vi "WinCI Get Default Provider.vi"(8 "error in (no error)":errorcluster) -> (0 "error out":errorcluster, 2 "default provider":string)   [LabVIEW 2017, in "NI_SCC_WinCI.lvlib"]
uses:
  <vilib>/SourceControl/Providers/WinCI/NI_SCC_WinCI.lvlib
  <vilib>/registry/registry.llb/Registry RtKey.ctl
  <vilib>/registry/registry.llb/Registry SAM.ctl
  <vilib>/registry/registry.llb/Read Registry Value Simple STR.vi
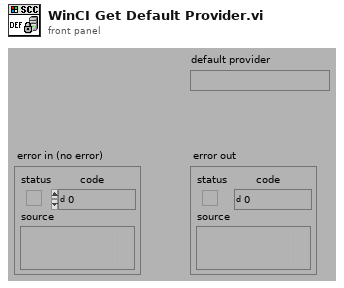
[diagram p1: front panel]
types:
  T1 = typedef "Registry SAM.ctl" = enum32{"KEY_QUERY_VALUE", "KEY_SET_VALUE", "KEY_CREATE_SUB_KEY", "KEY_ENUMERATE_SUB_KEYS", "KEY_NOTIFY", "KEY_CREATE_LINK", "KEY_READ", "KEY_WRITE", "KEY_ALL_ACCESS", "KEY_READ | KEY_WRITE"}
  T2 = typedef "Registry RtKey.ctl" = enum32{"HKEY_CLASSES_ROOT", "HKEY_CURRENT_USER", "HKEY_LOCAL_MACHINE", "HKEY_USERS", "HKEY_PERFORMANCE_DATA", "HKEY_CURRENT_CONFIG", "HKEY_DYN_DATA"}
  T3 = typedef "Registry refnum.ctl" = refnum<k1>
  T4 = cluster{"numValues":i32, "maxValueNameLen":i32, "maxValueDataLen":i32}
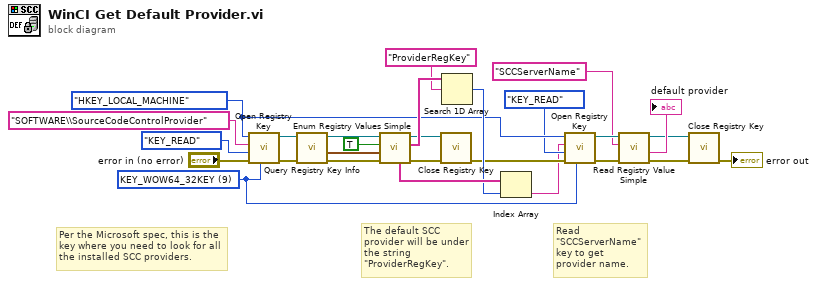
[diagram p0: block diagram]
diagram:
  w1 = u16 9 items=["DEFAULT"=0, "KEY_WOW64_64KEY"=8, "KEY_WOW64_32KEY"=9] ("alternate registry view mask")
  w9 = Registry_RtKey."HKEY_LOCAL_MACHINE" ("root key (HKEY_LOCAL_MACHINE)")
  # "Read \"SCCServerName\" key to get provider name."
  # "The default SCC provider will be under the string \"ProviderRegKey\"."
  # "Per the Microsoft spec, this is the key where you need to look for all the installed SCC providers."
  n1 = call <vilib>:"Open Registry Key.vi"("registry view"=w1, "error in (no error)"="error in (no error)", "security access mask (KEY_READ | KEY_WRITE)"=Registry_SAM."KEY_READ", "subkey"="SOFTWARE\\SourceCodeControlProvider", "root key (HKEY_LOCAL_MACHINE)"=w9) -> ("error out"=w20:errorcluster, "refnum out"=w19:T3)  [unwired: 5 out]
  n2 = call <vilib>:"Query Registry Key Info.vi"("error in (no error)"=w20, "refnum"=w19) -> ("error out"=w22:errorcluster, "value info"=w23:T4, "refnum out"=w21:T3)  [unwired: 7 out]
  n3 = call <vilib>:"Enum Registry Values Simple.vi"("error in (no error)"=w22, "value info"=w23, "retrieve data? (F)"=TRUE, "refnum"=w21) -> ("error out"=w11:errorcluster, "values"=w17:string[], "refnum out"=w12:T3, "String/Binary data"=w15:string[])  [unwired: 4 out]
  n4 = call <vilib>:"Close Registry Key.vi"("error in (no error)"=w11, "refnum"=w12) -> ("error out"=w10:errorcluster)  [unwired: 5 out]
  n5 = Search 1D Array(1D array=w17, element="ProviderRegKey" ("subkey")) -> (index of element=w14:i32)  [unwired: 1 out]
  n6 = Index Array(array=w15, index=w14) -> (element=w3:string)
  n7 = call <vilib>:"Open Registry Key.vi"("registry view"=w1, "error in (no error)"=w10, "security access mask (KEY_READ | KEY_WRITE)"=Registry_SAM."KEY_READ", "subkey"=w3, "root key (HKEY_LOCAL_MACHINE)"=w9) -> ("error out"=w6:errorcluster, "refnum out"=w7:T3)  [unwired: 5 out]
  n8 = call-poly <vilib>:"Read Registry Value Simple.vi"("error in (no error)"=w6, "value"="SCCServerName" ("subkey"), "refnum"=w7) -> ("error out"=w4:errorcluster, "String/Binary data"=→"default provider":string, "refnum out"=w5:T3)  [unwired: 1 in, 3 out]
  n9 = call <vilib>:"Close Registry Key.vi"("error in (no error)"=w4, "refnum"=w5) -> ("error out"=→"error out":errorcluster)  [unwired: 5 out]
